vi "Custom Freq Multiplier 2.vi"(7 "Number of pulses":u32=5) -> (0 "DO State":bool, 1 "Toggle Iterations":u32, 2 "Time elapsed (ticks)":u32, 3 "FIFO Read Timed Out?":bool)   [LabVIEW 2014]
doc: "This VI is a consumer for the FIFO. The FIFO will return the dt needed for pulse high time and low time.\n\nThis VI has 2 functions.\nIf FIFO element is pos, it will generate pulse according to dt from FIFO and \"Number of pulse\" input.\nIf FIFO element is neg, it will delay according to dt from FIFO."
uses:
  Custom Pulse 2.ctl
  <vilib>/rvi/Emulation/niFpgaEmulationIsFPGAContextNoSignature.vi
  <vilib>/rvi/Emulation/niFpgaSctlEmulationGetInTimedLoop.vi
  <vilib>/rvi/errors/niFpgaSetErrorForExecOnDevCompSimple.vi
  <vilib>/rvi/eio/common/nirviEmuReportErrorAndStop.vi
  <vilib>/rvi/DataTransferAndStorage/Container/Common/niFpgaContainerGetUniqueNameForEmu.vi
  <vilib>/rvi/FIFO/Fifo_Resource/nirvififoEmulationSetSize.vi
  <vilib>/rvi/FIFO/Fifo_Resource/nirviFifoEmulationQueueMgr.vi
  <instcachedir>/0/nirviFifoEmulationQueueMgr_E5CAEC123FF24DC58D834DCA3CDAA9B5.lvgen/nirviFifoEmulationQueueMgr_E5CAEC123FF24DC58D834DCA3CDAA9B5_004.vi
  <vilib>/rvi/FIFO/Fifo_Resource/nirvififoEmulationCreateLock.vi
  <vilib>/rvi/Emulation/niFpgaProcessEmulError.vi
  <vilib>/rvi/FIFO/Fifo_Resource/nirvififoEmulationObtainLock.vi
  <vilib>/rvi/FIFO/Fifo_Resource/nirvififoEmulationReleaseLock.vi
  <vilib>/rvi/occurrence/nirviWaitOnOccurrenceBase.vi
  <vilib>/rvi/errors/nirviReportUnexpectedCaseInternalError.vi
  <vilib>/rvi/errors/nirviReportUnexpectedCaseInternalError (U32).vi
  <vilib>/rvi/DataTransferAndStorage/Container/XNode/niFpgaContainer.xnode
  <vilib>/rvi/FIFO/Fifo_Resource/nirvififoEmulationRead.vi
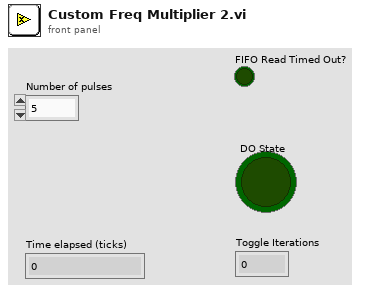
[diagram p1: front panel]
types:
  T1 = typedef "Custom Pulse 2.ctl" = enum16{"Idle", "Processing", "Delay"}
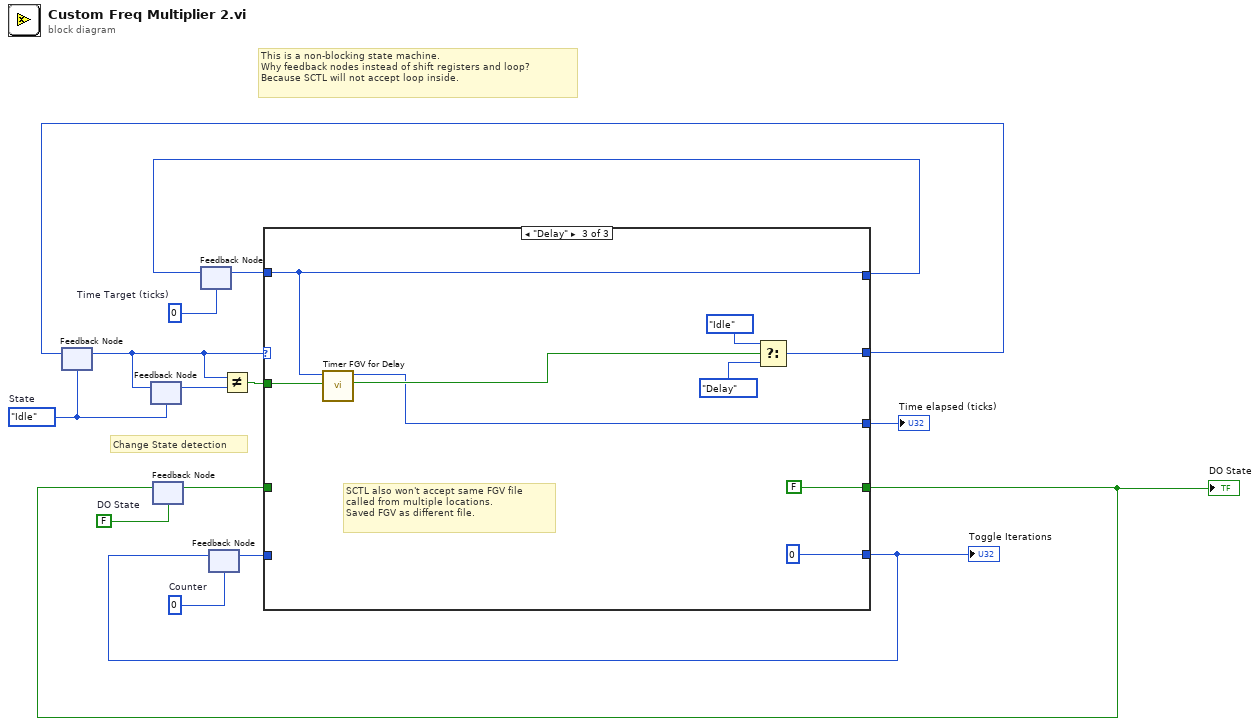
[diagram p0: block diagram]
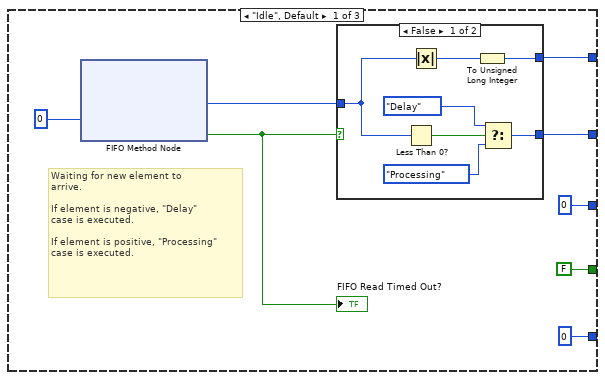
[diagram p2: hidden frame]
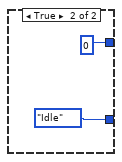
[diagram p3: hidden frame]
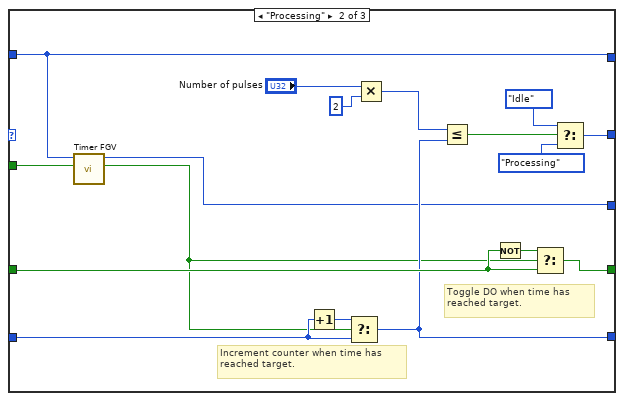
[diagram p4: hidden frame]
diagram:
  w5 = Custom_Pulse_2."Idle"  # State
  w7 = FALSE  # DO State
  w8 = u32 0  # Counter
  w9 = u32 0  # Time Target (ticks)
  # "This is a non-blocking state machine.\nWhy feedback nodes instead of shift registers and loop?\nBecause SCTL will not accept loop inside."
  # "Change State detection"
  n1 = feedback #1(w5) -> (w4:T1)
  n2 = feedback #2(w5) -> (w3:T1)
  n3 = feedback-in #2(w4) -> ()
  n4 = feedback #3(w7) -> (w12:bool)
  n5 = feedback #4(w9) -> (w15:u32)
  n6 = feedback #5(w8) -> (w14:u32)
  n7 = Not Equal?(x=w4, y=w3) -> (x != y?=w2:bool)
  n8 = case shown="\"Delay\"" w4 {
    tunnel: [w16 w37 w57] -> w10
    tunnel: [w19 w43 w54] -> w6
    tunnel: w15 -> [_ w37 w57]
    tunnel: w14 -> [_ w40 _]
    tunnel: [u32 0 w38 u32 0 ("Counter")] -> w13
    tunnel: w12 -> [_ w47 _]
    tunnel: [FALSE ("DO State") w46 FALSE ("DO State")] -> w11
    tunnel: w2 -> [_ w34 w58]
    tunnel: [u32 0 ("Time elapsed (ticks)") w33 w50] -> w1
    frame "Idle", Default {
      # "Waiting for new element to\narrive.\n\nIf element is negative, \"Delay\"\ncase is executed.\n\nIf element is positive, \"Processing\"\ncase is executed."
      n9 = xnode ("FIFO Method Node")("Timeout"=0) -> ("Element"=w17:i32, "Timed Out?"=w20:bool)  [unwired: 1 in, 1 out]
      "FIFO Read Timed Out?" <- w20
      n10 = case shown="False" w20 {
        tunnel: [w30 Custom_Pulse_2."Idle"] -> w19
        tunnel: w17 -> [w26 _]
        tunnel: [w24 u32 0 ("Element")] -> w16
        frame False {
          n11 = Less Than 0?(x=w26) -> (x < 0?=w27:bool)
          n12 = Absolute Value(x=w26) -> (abs(x)=w25:i32)
          n13 = To Unsigned Long Integer(number=w25) -> (unsigned 32bit integer=w24:u32)
          n14 = Select(t=Custom_Pulse_2."Delay", s=w27, f=Custom_Pulse_2."Processing") -> (s? t:f=w30:T1)
        }
        frame True {
        }
      }
    }
    frame "Processing" {
      # "Increment counter when time has\nreached target."
      # "Toggle DO when time has\nreached target."
      n15 = call "Timer FGV.vi"("Reset"=w34, "Time Target (ticks)"=w37) -> ("Time Reached?"=w36:bool, "Time elapsed (ticks)"=w33:u32)  [unwired: 8 in]
      n16 = Increment(x=w40) -> (x+1=w49:u32)
      n17 = Select(t=w49, s=w36, f=w40) -> (s? t:f=w38:u32)
      n18 = Multiply(x="Number of pulses", y=u32 2) -> (x*y=w39:u32)
      n19 = Less Or Equal?(x=w39, y=w38) -> (x <= y?=w42:bool)
      n20 = Not(x=w47) -> (.not. x?=w48:bool)
      n21 = Select(t=w48, s=w36, f=w47) -> (s? t:f=w46:bool)
      n22 = Select(t=Custom_Pulse_2."Idle", s=w42, f=Custom_Pulse_2."Processing") -> (s? t:f=w43:T1)
    }
    frame "Delay" {
      # "SCTL also won't accept same FGV file\ncalled from multiple locations.\nSaved FGV as different file."
      n23 = call "Timer FGV for Delay.vi"("Reset"=w58, "Time Target (ticks)"=w57) -> ("Time Reached?"=w53:bool, "Time elapsed (ticks)"=w50:u32)  [unwired: 8 in]
      n24 = Select(t=Custom_Pulse_2."Idle", s=w53, f=Custom_Pulse_2."Delay") -> (s? t:f=w54:T1)
    }
  }
  "Toggle Iterations" <- w13
  "DO State" <- w11
  "Time elapsed (ticks)" <- w1
  n25 = feedback-in #1(w6) -> ()
  n26 = feedback-in #3(w11) -> ()
  n27 = feedback-in #4(w10) -> ()
  n28 = feedback-in #5(w13) -> ()
